vi "Set Buffer Size.vi"(10 "Buffer Size":u32=32000, 11 "Messaging Buffer in":refnum<class "Message Buffer.lvclass">) -> (3 "Messaging Buffer out":refnum<class "Message Buffer.lvclass">)   [LabVIEW 2024, in "PCAN.lvlib" / "Message Buffer.lvclass"]
uses:
  Message Buffer.lvclass
  Message Buffer.lvclass/Message Buffer.ctl
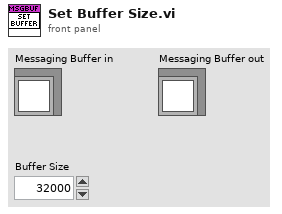
[diagram p1: front panel]
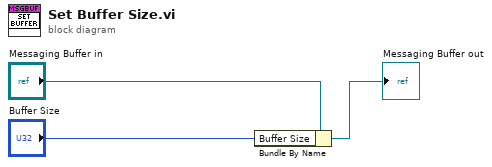
[diagram p0: block diagram]
diagram:
  n1 = Bundle By Name(cluster="Messaging Buffer in", "Buffer Size"="Buffer Size") -> (→"Messaging Buffer out":refnum<class "Message Buffer.lvclass">)
